vi "ReportEnd_A131258.vi"(6 "文件重命名":bool, 8 "error in (no error)":errorcluster caption="错误输入（无错误）", 10 "文件名称":string, 11 "report in":refnum<class "NI_report.lvclass"> caption="报表输入") -> (0 "error out":errorcluster caption="错误输出")   [LabVIEW 2020]
uses:
  <vilib>/Utility/NIReport.llb/NI_report.lvclass
  Global_Variable/Global.vi
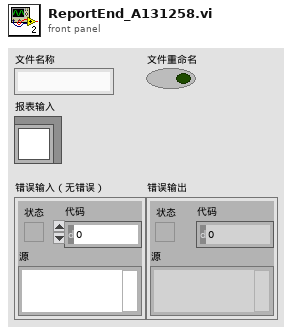
[diagram p1: front panel]
types:
  T1 = cluster{"Italic":enum16{"Italic Unchanged", "Italic On", "Italic Off"}, "Strike Through":enum16{"Strike Through Unchanged", "Strike Through On", "Strike Through Off"}, "Underline":enum16{"Underline Unchanged", "Underline On", "Underline Off"}, "Bold":enum16{"Bold Unchanged", "Bold On", "Bold Off"}}
  T2 = cluster{"Charset (-1)":i16, "Weight (-1)":i16, "Name":string, "Size":string}
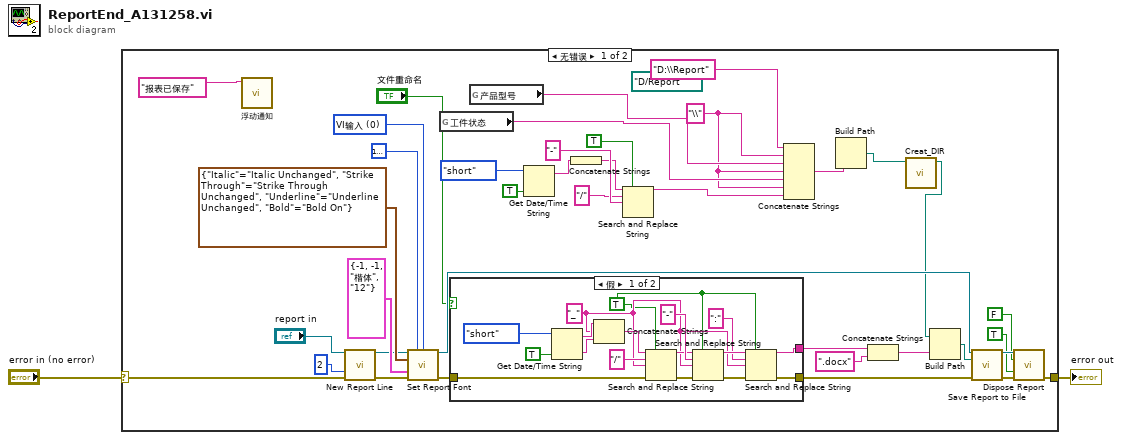
[diagram p0: block diagram]
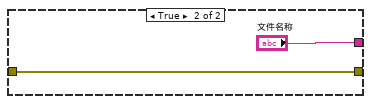
[diagram p2: hidden frame]
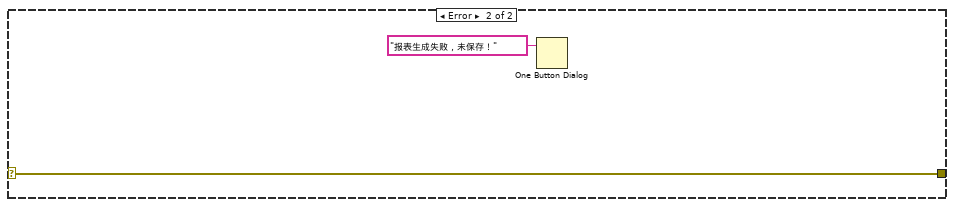
[diagram p3: hidden frame]
diagram:
  n1 = case shown="无错误" "error in (no error)" {
    selector: "error in (no error)" -> [w24 w61]
    tunnel: [w23 w61] -> w1
    frame No Error {
      w4 = "\\" ("搜索字符串")
      w34 = u16 0 items=["VI输入", "字体对话框"] ("font settings source")
      (unwired) path "D:/Report" ("report file path")
      n2 = call "浮动通知.vi"("通知内容"="报表已保存") -> ()  [unwired: 11 in]
      n3 = call-dynamic "New Report Line.vi"("report in"="report in", "number of lines (1)"=2, "error in (no error)"=w24) -> ("report out"=w31:refnum<class "NI_report.lvclass">, "error out"=w30:errorcluster)  [unwired: 11 in]
      n4 = call-dynamic "Set Report Font.vi"("report in"=w31, "text color (unchanged)"=u32 16777224, "font settings source (VI Inputs)"=w34, "text options"=T1 {"Italic"=enum."Italic Unchanged", "Strike Through"=enum."Strike Through Unchanged", "Underline"=enum."Underline Unchanged", "Bold"=enum."Bold On"}, "font settings"=T2 {"Charset (-1)"=-1, "Weight (-1)"=-1, "Name"="楷体", "Size"="12"}, "error in (no error)"=w30) -> ("report out"=w27:refnum<class "NI_report.lvclass">, "error out"=w26:errorcluster)  [unwired: 7 in, 1 out]
      n5 = global read "追溯全部变量.vi" "工件状态"() -> (w5:string)
      n6 = case shown="假" "文件重命名" {
        tunnel: [w52 "文件名称"] -> w21
        tunnel: w26 -> [w44 w58]
        tunnel: [w41 w58] -> w25
        frame False {
          w46 = TRUE ("替换全部？(F)")
          w47 = "_" ("替换字符串(\"\")")
          n7 = Get Date/Time String(date format (0)=enum16{"short", "long", "abbreviated"}."short" ("日期格式(0)"), want seconds? (F)=TRUE ("需要秒？(F)")) -> (date string=w57:string, time string=w53:string)  [unwired: 1 in]
          n8 = Concatenate Strings(w57, w47, w53) -> (w50:string)
          n9 = Search and Replace String(replace all?=w46, input string=w50, search string="/" ("搜索字符串"), replace string=w47, error in=w44) -> (result string=w49:string, error out=w43:errorcluster)  [unwired: 3 in, 2 out]
          n10 = Search and Replace String(replace all?=w46, input string=w49, search string="-" ("搜索字符串"), replace string=w47, error in=w43) -> (result string=w55:string, error out=w42:errorcluster)  [unwired: 3 in, 2 out]
          n11 = Search and Replace String(replace all?=w46, input string=w55, search string=":" ("搜索字符串"), replace string=w47, error in=w42) -> (result string=w52:string, error out=w41:errorcluster)  [unwired: 3 in, 2 out]
        }
        frame True {
        }
      }
      n12 = global read "Global.vi" "产品型号"() -> (w6:string)
      n13 = Get Date/Time String(date format (0)=enum16{"short", "long", "abbreviated"}."short" ("日期格式(0)"), want seconds? (F)=TRUE ("需要秒？(F)")) -> (date string=w12:string)  [unwired: 1 in, 1 out]
      n14 = Concatenate Strings(w12) -> (w14:string)
      n15 = Search and Replace String(replace all?=TRUE ("替换全部？(F)"), input string=w14, search string="/" ("搜索字符串"), replace string="-" ("替换字符串(\"\")")) -> (result string=w7:string)  [unwired: 4 in, 3 out]
      n16 = Concatenate Strings("D:\\Report" ("搜索字符串"), w4, w6, w4, w5, w4, w7) -> (w11:string)
      n17 = Build Path(name or relative path=w11) -> (appended path=w10:path)  [unwired: 1 in]
      n18 = Concatenate Strings(w21, ".docx" ("字符串")) -> (w20:string)
      n19 = call "Creat_DIR.vi"("path"=w10) -> ("created path"=w9:path)  [unwired: 10 in]
      n20 = Build Path(base path=w9, name or relative path=w20) -> (appended path=w36:path)
      n21 = call-dynamic "Save Report to File.vi"("report in"=w27, "report file path"=w36, "error in (no error)"=w25) -> ("report out"=w40:refnum<class "NI_report.lvclass">, "error out"=w39:errorcluster)  [unwired: 11 in]
      n22 = call-dynamic "Dispose Report.vi"("report in"=w40, "wait until printing completed? (T)"=FALSE, "save changes? (F)"=TRUE, "error in (no error)"=w39) -> ("error out"=w23:errorcluster)  [unwired: 11 in]
    }
    frame Error {
      n23 = One Button Dialog(message="报表生成失败，未保存！" ("消息")) -> ()  [unwired: 1 in, 1 out]
    }
  }
  "error out" <- w1
